vi "AVS_GetLambda.vi"(0 "a_hDevice":i32, 11 "a_pWaveLength":dbl[](array[numeric])) -> (4 "Output Value":i32, 15 "a_pWaveLength":dbl[](array[numeric]))   [LabVIEW 2014, in "AvaSpec.lvlib" / "Avantes Spectrometer Functions.lvlib"]
uses:
  Avantes Spectrometer Functions.lvlib
  AS5216.dll
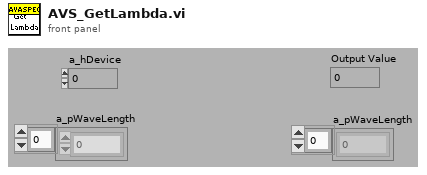
[diagram p1: front panel]
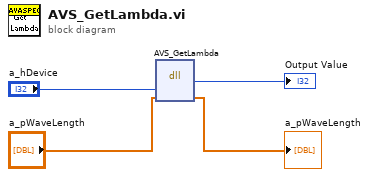
[diagram p0: block diagram]
diagram:
  n1 = dll-call lib="C:/Users/Daniel/Dropbox/CLTC/avantesSpectrometer/Libraries/AS-5216-DLL/polling_mc/AS5216.dll" fn="AVS_GetLambda"("a_hDevice"="a_hDevice", "a_pWaveLength"="a_pWaveLength") -> (→"Output Value":i32, "a_pWaveLength"=→"a_pWaveLength":dbl[])  [unwired: 4 in, 2 out]
